vi "Streamlined FPGA--smooth variable window.vi"() -> ()   [LabVIEW 2009]
uses:
  <vilib>/eio/EIONode/EIONode.xnode
  <vilib>/rvi/eio/nirviEIOImplementation/nirviEIOImplementation.xnode
  <vilib>/rvi/eio/common/nirviEmuTemplateMethod_noerrors.vi
  <vilib>/rvi/eio/common/nirviEmuClasses.ctl
  Instance           3 24Saved   Streamlined FPGA .vi
  Instance           4 24Saved   Streamlined FPGA .vi
  Instance           5 24Saved   Streamlined FPGA .vi
  Instance           2 24Saved   Streamlined FPGA .vi
  <vilib>/rvi/DataTransferAndStorage/Container/XNode/niFpgaContainer.xnode
  <vilib>/rvi/interface/RandomDataEmulation/niFpgaRandomDataHandleErrors.vi
  <vilib>/rvi/interface/RandomDataEmulation/nirviRandomDataFPGAFIFO.vi
  <vilib>/rvi/DataTransferAndStorage/Container/Common/niFpgaContainerMethod.ctl
  <vilib>/rvi/DataTransferAndStorage/Container/Common/niFpgaTransferTypeControl.ctl
panel:
  in  "window size":i32
  in  "smooth":bool
  in  "Rec2 Ymin":i32
  in  "Rec2 Xmin":i32
  in  "Rec1 Ymin":i32
  in  "Rec1 Xmin":i32
  in  "Rec2 Ymax":i32
  in  "Rec1 Ymax":i32
  in  "Rec2 Xmax":i32
  in  "Rec1 Xmax":i32
  out "sort!":bool
  in  "Maximum Width":i16
  in  "Maximum Height":i16
  in  "trigger on all":bool
  out "sort pulse":i16
  in  "Baselines":i16[](array[numeric])=[0, 0, 0, 0]
  in  "Sb":i8(ring)=1 items=["PMT1", "PMT2", "PMT3", "PMT4"]
  in  "Sa":i8(ring) items=["PMT1", "PMT2", "PMT3", "PMT4"]
  in  "Sort Case":i8(ring)=1 items=["FP", "Magnitude"]
  out "Full 2":bool
  in  "sort?":bool
  out "Drop counter":u32
  out "sort counter":u32
  in  "PMT to detect drops on":u8
  in  "Minimum Height":i16
  in  "Minimum Width":i16
  in  "Ticks between acquires (Ticks)":u32=200
  in  "Gain 1":i16(slide) scale=-32767.0..32767.0
  in  "Gain 2":i16(slide) scale=-32767.0..32767.0
  in  "Gain 3":i16(slide) scale=-32767.0..32767.0
  in  "Gain 4":i16(slide) scale=-32767.0..32767.0
  in  "amplitude":i16
  in  "1/Frequency \n(ticks)":u32
  in  "Burst \nCycles":i32
  in  "delay [us]":u32=20 min=1 max=8000
  # "Acquisition and Detection"
  # "FP and Sorting Parameters"
  # "Sorting Pulse\nGenerator"
  # "Events"
  # "PMT Controls"
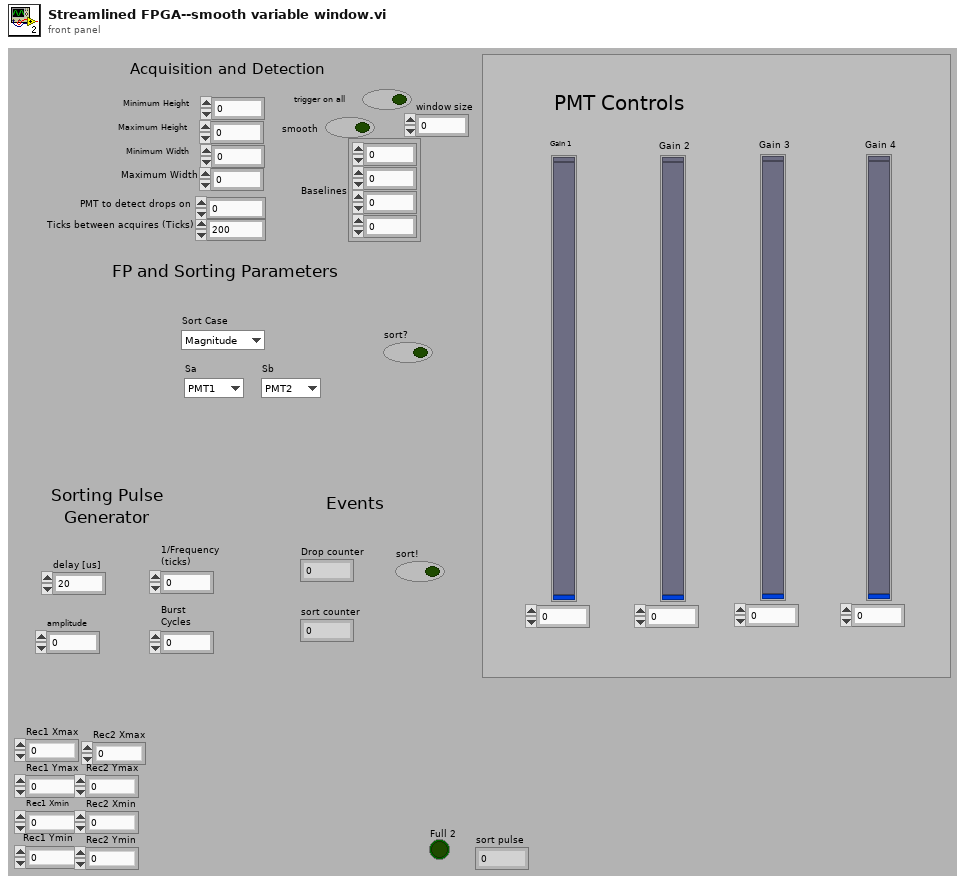
[diagram p1: front panel]
types:
  T1 = typedef "nirviEmuClasses.ctl" = enum16{"IO Read", "IO Write", "Method", "Property Read", "Property Write"}
  T2 = cluster{i32[], i32[], i32[], i32[], i32[], i32[], i32[], i32[]}
  T3 = typedef "niFpgaContainerMethod.ctl" = enum16{"Write", "Read", "Clear", "Get Number of Elements to Write", "Get Number of Elements to Read", "Enable", "Disable", "Flush and Disable", "Get Stream State"}
  T4 = typedef "niFpgaTransferTypeControl.ctl" = enum16{"Target-Scoped", "Host to Target - DMA", "Target to Host - DMA", "Peer to Peer Reader", "Peer to Peer Writer", "Bidirectional"}
  T5 = cluster{"Rec1 Xmax":i32, "Rec1 Ymax":i32, "Rec1 Xmin":i32, "Rec1 Ymin":i32, "Rec2 Xmax":i32, "Rec2 Ymax":i32, "Rec2 Xmin":i32, "Rec2 Ymin":i32}
  T6 = cluster{bool, "max":i16[], "sum":i32[], "time inside":i32, "time outside":i32, "timeoutside-1":i32}
  T7 = cluster{"maxes":i16[], "sums":i32[], "time inside":i32, "time outside":i32}
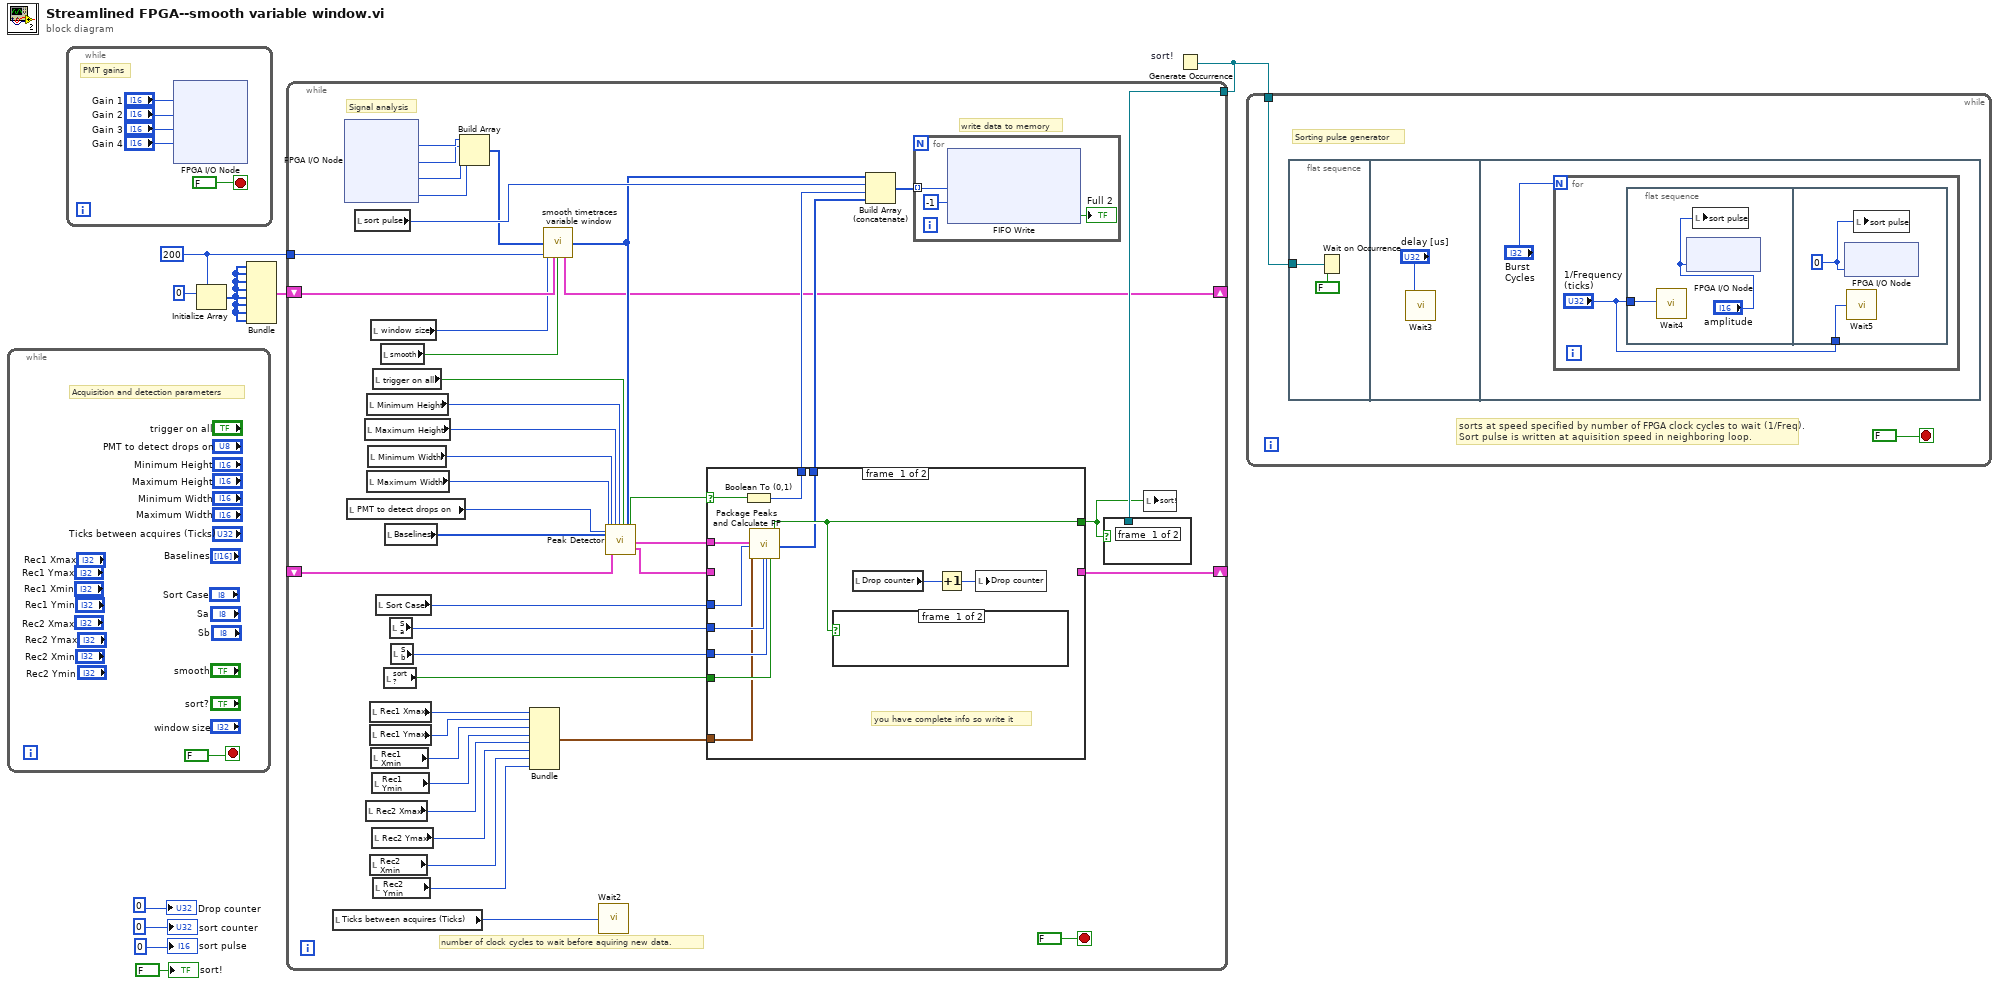
[diagram p0: block diagram]
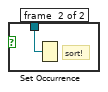
[diagram p2: hidden frame]
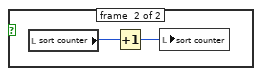
[diagram p3: hidden frame]
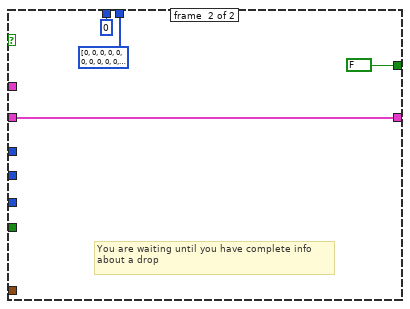
[diagram p4: hidden frame]
diagram:
  w1 = 200 ("dimension size")
  n1 = while {
    stop <- FALSE stop-if-true
    # "Acquisition and detection parameters"
  }
  n2 = while {
    stop <- FALSE stop-if-true
    # "PMT gains"
    n3 = xnode "FPGA I/O Node"("AO0"="Gain 1", "AO1"="Gain 2", "AO2"="Gain 3", "AO3"="Gain 4") -> ()  [unwired: 4 in, 4 out]
  }
  n4 = Initialize Array(0 ("element"), w1) -> (w4:i32[])
  n5 = Bundle(w4, w4, w4, w4, w4, w4, w4, w4) -> (w2:T2)  [unwired: 1 in]
  n6 = Generate Occurrence "sort!"() -> (w9:refnum<k4>)
  n7 = while {
    shift-right: [w102] -> _
    shift-left: _ -> [w89]
    tunnel: w9 -> [w87]
    shift-right: [w63] -> _
    shift-left: w2 -> [w64]
    tunnel: w1 -> [w62]
    stop <- FALSE stop-if-true
    # "number of clock cycles to wait before aquiring new data."
    # "Signal analysis"
    # "write data to memory"
    n8 = local read "Ticks between acquires (Ticks)"() -> (w97:u32)
    n9 = xnode "FPGA I/O Node"() -> ("AI0"=w101:i16, "AI1"=w100:i16, "AI2"=w99:i16, "AI3"=w98:i16)  [unwired: 4 in, 4 out]
    n10 = local read "PMT to detect drops on"() -> (w79:u8)
    n11 = local read "sort pulse"() -> (w86:i16)
    n12 = local read "Maximum Height"() -> (w82:i16)
    n13 = local read "Rec2 Xmax"() -> (w71:i32)
    n14 = local read "Minimum Height"() -> (w83:i16)
    n15 = local read "Maximum Width"() -> (w80:i16)
    n16 = local read "Minimum Width"() -> (w81:i16)
    n17 = local read "Rec1 Xmax"() -> (w75:i32)
    n18 = local read "Rec1 Ymax"() -> (w74:i32)
    n19 = local read "Rec2 Xmin"() -> (w69:i32)
    n20 = local read "window size"() -> (w61:i32)
    n21 = local read "Rec1 Xmin"() -> (w73:i32)
    n22 = local read "Rec1 Ymin"() -> (w72:i32)
    n23 = local read "Rec2 Ymax"() -> (w70:i32)
    n24 = local read "trigger on all"() -> (w88:bool)
    n25 = local read "Rec2 Ymin"() -> (w68:i32)
    n26 = local read "Sort Case"() -> (w96:i8)
    n27 = local read "smooth"() -> (w60:bool)
    n28 = local read "sort?"() -> (w93:bool)
    n29 = local read "Baselines"() -> (w78:i16[])
    n30 = local read "Sa"() -> (w95:i8)
    n31 = local read "Sb"() -> (w94:i8)
    n32 = Build Array(w101, w100, w99, w98) -> (w65:i16[])
    n33 = Bundle("Rec1 Xmax"=w75, "Rec1 Ymax"=w74, "Rec1 Xmin"=w73, "Rec1 Ymin"=w72, "Rec2 Xmax"=w71, "Rec2 Ymax"=w70, "Rec2 Xmin"=w69, "Rec2 Ymin"=w68) -> (w67:T5)  [unwired: 1 in]
    n34 = call "smooth timetraces variable window.vi"("smooth"=w60, "PMT data"=w65, "window size"=w61, "max window size"=w62, "sums in"=w64) -> ("smoothed data"=w66:i16[], "sums out"=w63:T2)  [unwired: 9 in]
    n35 = call "Wait2"("Count(Ticks)"=w97) -> ()  [unwired: 1 out]
    n36 = call "Peak Detector.vi"("Maximum Width"=w80, "PMT to trigger on (0,1,2,3)"=w79, "Baselines"=w78, "Minimum Width"=w81, "shifts in"=w89, "Maximum Height"=w82, "Minimum Height"=w83, "trigger on all"=w88, "s1,s2,s3,s4"=w66) -> ("peak complete?"=w92:bool, "shifts out"=w90:T6, "peaks data"=w91:T7)  [unwired: 16 in]
    n37 = case shown="True" w92 {
      selector: w92 -> [w214 _]
      tunnel: [_ w225] -> w102
      tunnel: [w212 FALSE ("sort!")] -> w77
      tunnel: w96 -> [w210 _]
      tunnel: w95 -> [w218 _]
      tunnel: w94 -> [w217 _]
      tunnel: w93 -> [w216 _]
      tunnel: w90 -> [_ w225]
      tunnel: w91 -> [w215 _]
      tunnel: [w213 i16 0] -> w84
      tunnel: [w211 i32[] [0, 0, 0, 0, 0, 0, 0, 0, 0, 0, 0, 0] ("M1,M2,M3,M4,S1,S2,S3,S4,Tin,Tout,FP")] -> w76
      tunnel: w67 -> [w209 _]
      frame #0 {
        # "you have complete info so write it"
        n38 = Boolean To (0,1)(Boolean=w214) -> (0, 1=w213:i16)
        n39 = call "Package Peaks and Calculate FP.vi"("peaks data"=w215, "Sort Case"=w210, "Rectangle Positions"=w209, "Sa"=w218, "Sb"=w217, "sort?"=w216) -> ("sort!"=w212:bool, "M1,M2,M3,M4,S1,S2,S3,S4,Tin,Tout,FP,Sort?"=w211:i32[])  [unwired: 14 in, 6 out]
        n40 = case shown="True" w212 {
          frame #0 {
          }
          frame #1 {
            n41 = local read "sort counter"() -> (w222:u32)
            n42 = Increment(x=w222) -> (x+1=w221:u32)
            n43 = local write "sort counter"(w221) -> ()
          }
        }
        n44 = local read "Drop counter"() -> (w220:u32)
        n45 = Increment(x=w220) -> (x+1=w219:u32)
        n46 = local write "Drop counter"(w219) -> ()
      }
      frame #1 {
        # "You are waiting until you have complete info about a drop"
      }
    }
    n47 = Build Array (concatenate)(w66, w86, w84, w76) -> (w85:i32[])
    n48 = for {
      tunnel: w85 -> [w107] mode=indexing
      n49 = xnode ("FIFO Write")("Element"=w107, "Timeout"=-1) -> ("Timed Out?"=→"Full 2":bool)  [unwired: 1 in, 1 out]
    }
    n50 = case shown="True" w77 {
      tunnel: w87 -> [_ w104]
      frame #0 {
      }
      frame #1 {
        # "sort!"
        n51 = Set Occurrence(w104) -> ()
      }
    }
    n52 = local write "sort!"(w77) -> ()
  }
  n53 = while {
    tunnel: w9 -> [w227]
    stop <- FALSE stop-if-true
    # "sorts at speed specified by number of FPGA clock cycles to wait (1/Freq).\nSort pulse is written at aquisition speed in neighboring loop."
    # "Sorting pulse generator"
    n54 = flat-sequence {
      tunnel: w227 -> [w229]
      frame #0 {
        n55 = Wait on Occurrence(1:FALSE ("ignore previous (T)"), 2:w229) -> ()  [unwired: 1 in, 1 out]
      }
      frame #1 {
        n56 = call "Wait3"("Count(uSec)"="delay [us]") -> ()  [unwired: 1 out]
      }
      frame #2 {
        n57 = for {
          N: "Burst \nCycles" -> [_]
          n58 = flat-sequence {
            tunnel: "1/Frequency \n(ticks)" -> [w235]
            tunnel: "1/Frequency \n(ticks)" -> [w248]
            frame #0 {
              n59 = call "Wait4"("Count(Ticks)"=w235) -> ()  [unwired: 1 out]
              n60 = xnode "FPGA I/O Node"("AO4"="amplitude") -> ()  [unwired: 1 in, 1 out]
              n61 = local write "sort pulse"("amplitude") -> ()
            }
            frame #1 {
              w247 = i16 0 ("sort pulse")
              n62 = xnode "FPGA I/O Node"("AO4"=w247) -> ()  [unwired: 1 in, 1 out]
              n63 = call "Wait5"("Count(Ticks)"=w248) -> ()  [unwired: 1 out]
              n64 = local write "sort pulse"(w247) -> ()
            }
          }
        }
      }
    }
  }
  "sort counter" <- u32 0 ("event counter")
  "Drop counter" <- u32 0 ("Drop counter")
  "sort pulse" <- i16 0 ("event counter")
  "sort!" <- FALSE ("sort!")
